vi "Increment String.vi"(9 "Numeric":u32, 10 "Input String":string, 11 "StringIncrement":refnum<class "StringIncrement.lvclass">) -> (1 "Incremented Numeric":u32, 2 "Incremented String":string)   [LabVIEW 2014, in "UniqueName.lvlib" / "StringIncrement.lvclass"]
uses:
  StringIncrement.lvclass
  StringIncrement.lvclass/StringIncrement.ctl
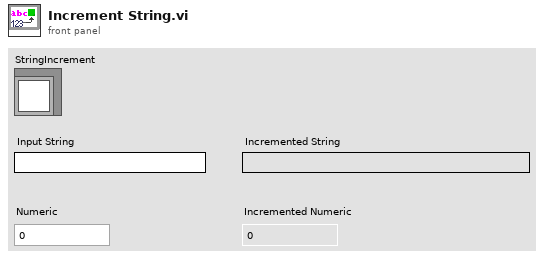
[diagram p1: front panel]
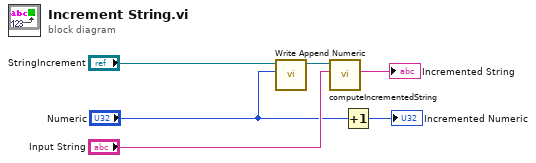
[diagram p0: block diagram]
diagram:
  n1 = call "Write Append Numeric.vi"("Append Numeric"="Numeric", "StringIncrement"="StringIncrement") -> ("StringIncrement out"=w4:refnum<class "StringIncrement.lvclass">)  [unwired: 9 in]
  n2 = call-dynamic "computeIncrementedString.vi"("Input String"="Input String", "StringIncrement"=w4) -> ("Incremented String"=→"Incremented String":string)  [unwired: 8 in, 1 out]
  n3 = Increment(x="Numeric") -> (x+1=→"Incremented Numeric":u32)
